vi "Set Run State Windows Pos.vi"(10 "Front Panel Window:Window Bounds":T1, 11 "reference":refnum<vi>) -> ()   [LabVIEW 2025, in "Full User Interface.lvlib"]
uses:
  Full User Interface.lvlib
  <vilib>/Utility/miscctls.llb/LVRectTypeDef.ctl
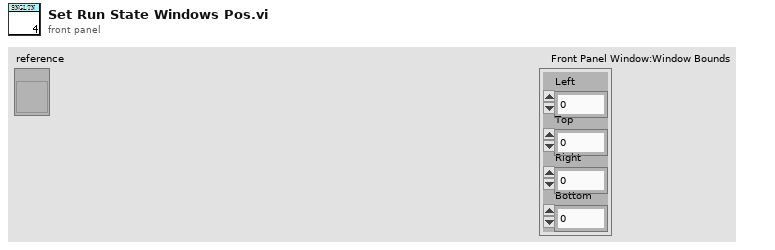
[diagram p1: front panel]
types:
  T1 = typedef "LVRectTypeDef.ctl" = cluster{"Left":i16, "Top":i16, "Right":i16, "Bottom":i16}
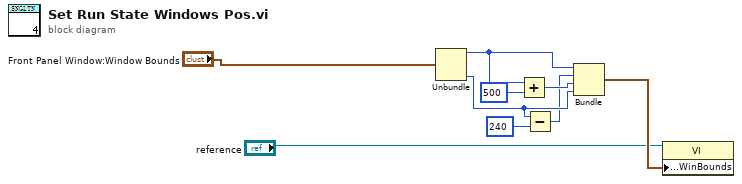
[diagram p0: block diagram]
diagram:
  n1 = Unbundle("Front Panel Window:Window Bounds") -> ("Left"=w8:i16, "Bottom"=w6:i16)  [unwired: 2 out]
  n2 = Add(x=w8, y=i16 500) -> (x+y=w7:i16)
  n3 = Subtract(x=w6, y=i16 240) -> (x-y=w4:i16)
  n4 = Bundle("Left"=w8, w4, w7, "Bottom"=w6) -> (w3:cluster{"Left":i16, i16, i16, "Bottom":i16})  [unwired: 1 in]
  n5 = property class="VI"(reference="reference", "Front Panel.WinBounds"=w3) -> ()  [unwired: 1 in, 2 out]
